vi "NI-DAQmxBase.vi"() -> (15 "error out":errorcluster)   [LabVIEW 2015]
uses:
  Globals/Meas_global.vi
  PWA/PWAtasksGLOBAL.vi
  <vilib>/_DAQmxBase/Internals/DAQmxBase Create Channel (AI-Voltage-Basic).vi
  <vilib>/_DAQmxBase/Internals/DAQmxBase Timing (Sample Clock).vi
  <vilib>/_DAQmxBase/Internals/DAQmxBase Read (Analog 2D DBL NChan NSamp).vi
  <resource>/objmgr/daqmx.rc
panel:
  out "AuditTrail":string[](array[string])
  out "input terminal configuration":i32(ring)=10106 items=["default"=-1, "RSE"=10083, "NRSE"=10078, "Differential"=10106, "Pseudodifferential"=12529]
  out "TotalSampPerChanAcquired":dbl=1024.0
  out "AvailSampPerChan":u32
  out "CurrReadPos":dbl=1024.0
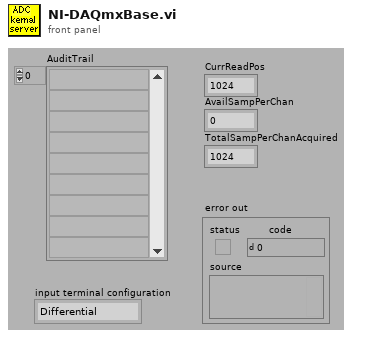
[diagram p1: front panel]
types:
  T1 = typedef "Ch_and_Spans.ctl" = cluster{"high limit (10V)":sgl, "low limit (-10V)":sgl, "Ch No":i16, "Var name":string, "Use Latest Calib":bool}
  T2 = typedef "LDA_Setup.ctl" = cluster{"dimensions":enum16{"1D", "2D"}, "Analogue Freq Multiplier":dbl}
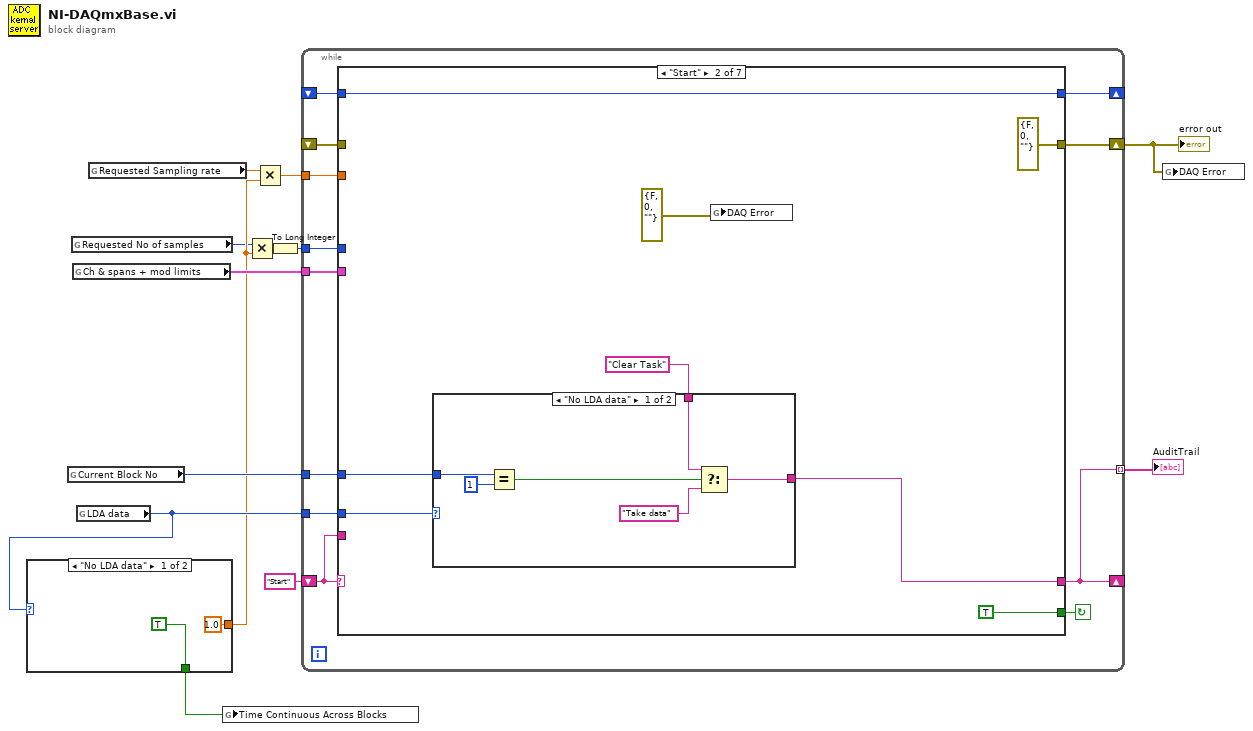
[diagram p0: block diagram]
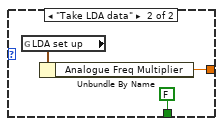
[diagram p2: hidden frame]
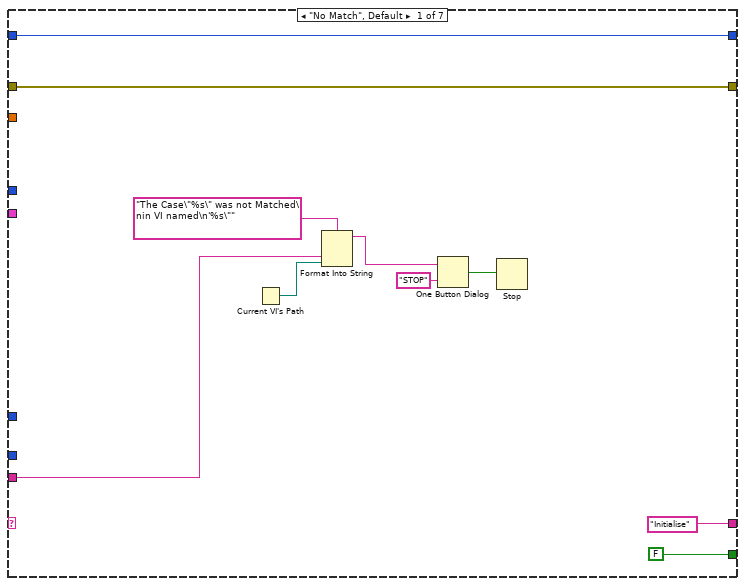
[diagram p3: hidden frame]
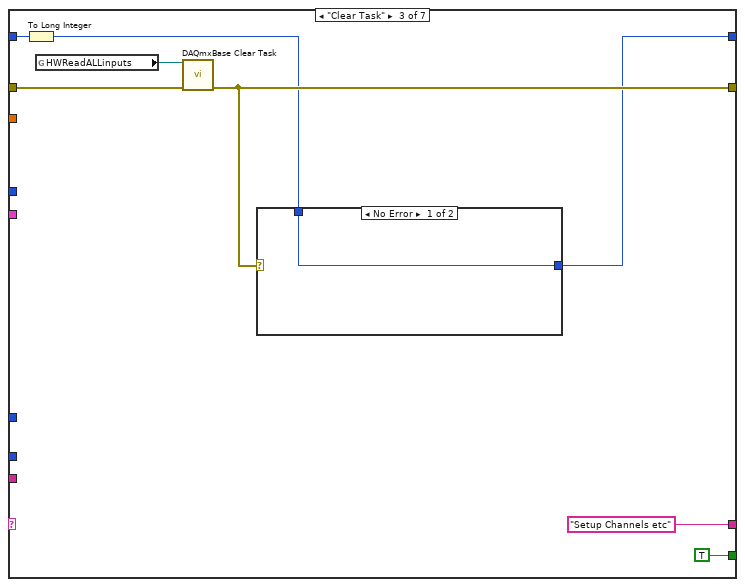
[diagram p5: hidden frame]
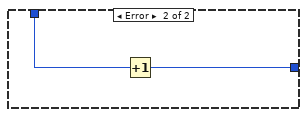
[diagram p6: hidden frame]
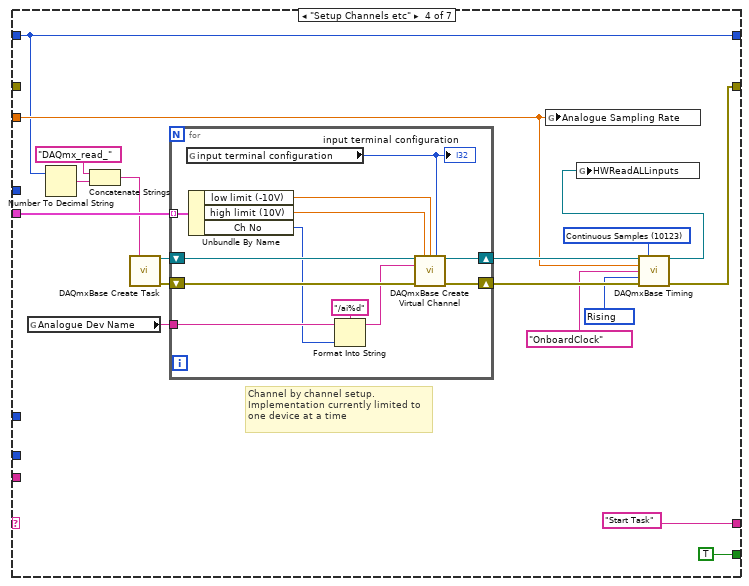
[diagram p7: hidden frame]
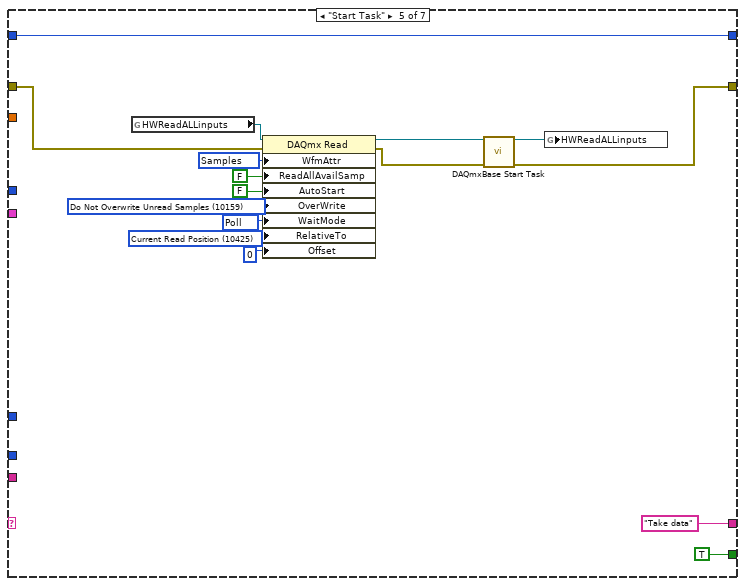
[diagram p8: hidden frame]
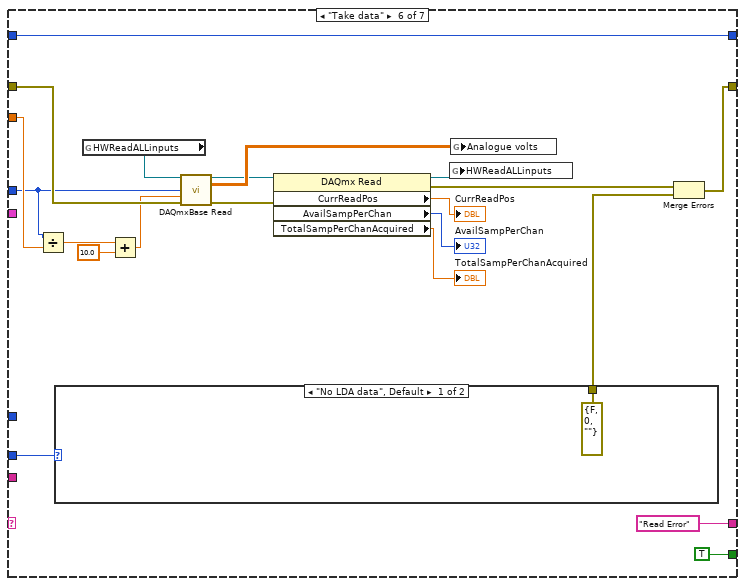
[diagram p9: hidden frame]
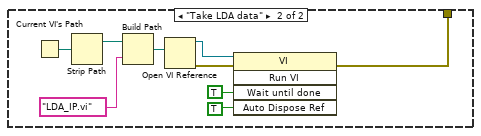
[diagram p10: hidden frame]
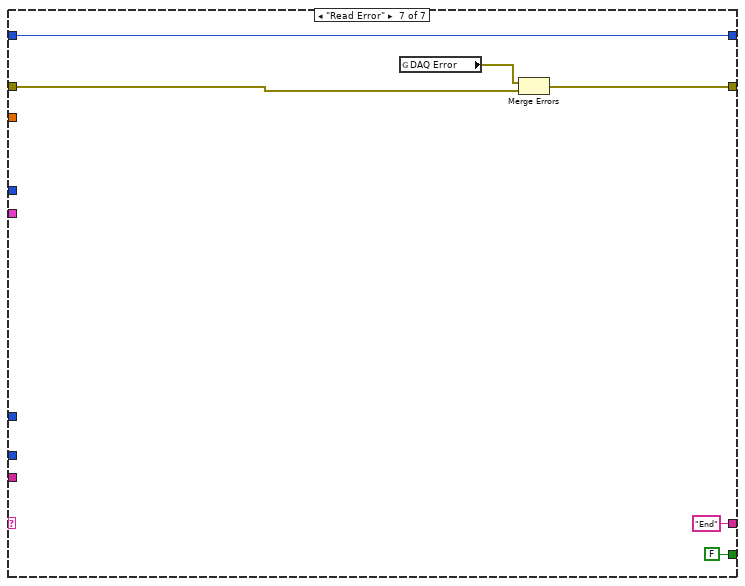
[diagram p11: hidden frame]
diagram:
  n1 = global read "Meas_global.vi" "Current Block No"() -> (w11:i32)
  n2 = global read "Meas_global.vi" "Requested No of samples"() -> (w1:i32)
  n3 = global read "Meas_global.vi" "Ch & spans + mod limits"() -> (w12:T1[])
  n4 = global read "Meas_global.vi" "LDA data"() -> (w9:enum16{"No LDA data", "Take LDA data"})
  n5 = case shown="\"No LDA data\"" w9 {
    tunnel: [1.0 ("Analogue Freq Multiplier") w17] -> w6
    tunnel: [TRUE ("Time Continuous across Blocks") FALSE ("Time Continuous across Blocks")] -> w2
    frame "No LDA data" {
    }
    frame "Take LDA data" {
      n6 = global read "Meas_global.vi" "LDA set up"() -> (w18:T2)
      n7 = Unbundle By Name(w18) -> ("Analogue Freq Multiplier"=w17:dbl)
    }
  }
  n8 = global read "Meas_global.vi" "Requested Sampling rate"() -> (w7:dbl)
  n9 = global write "Meas_global.vi" "Time Continuous Across Blocks"(w2) -> ()
  n10 = Multiply(x=w1, y=w6) -> (x*y=w8:dbl)
  n11 = Multiply(x=w7, y=w6) -> (x*y=w5:dbl)
  n12 = To Long Integer(number=w8) -> (32bit integer=w4:i32)
  n13 = while {
    shift-left: "Start" -> [w29]
    shift-right: [w19] -> _
    shift-right: [w23] -> w10
    shift-left: _ -> [w28]
    tunnel: w5 -> [w27]
    tunnel: w4 -> [w26]
    tunnel: w11 -> [w25]
    tunnel: w12 -> [w24]
    shift-right: [w22] -> _
    shift-left: _ -> [w21]
    tunnel: w9 -> [w20]
    tunnel: [w19] -> w3 mode=indexing
    stop <- w30 continue-if-true
    n14 = case shown="\"Start\"" w29 {
      tunnel: [FALSE TRUE TRUE TRUE TRUE TRUE FALSE] -> w30
      tunnel: ["Initialise" w46 "Setup Channels etc" "Start Task" "Take data" "Read Error" "End" ("f")] -> w19
      tunnel: w29 -> [w35 _ _ _ _ _ _]
      tunnel: [w32 errorcluster {"status"=FALSE, "code"=0, "source"=""} ("error out") w59 w78 w98 w115 w147] -> w23
      tunnel: w28 -> [w32 _ w60 _ w103 w133 w148]
      tunnel: w27 -> [_ _ _ w70 _ w123 _]
      tunnel: w26 -> [_ _ _ _ _ w114 _]
      tunnel: w25 -> [_ w43 _ _ _ _ _]
      tunnel: w24 -> [_ _ _ w77 _ _ _]
      tunnel: [w31 w45 w58 w69 w101 w124 w146] -> w22
      tunnel: w21 -> [w31 w45 w57 w69 w101 w124 w146]
      tunnel: w20 -> [_ w42 _ _ _ w118 _]
      frame "No Match", Default {
        n15 = Current VI's Path() -> (path=w34:path)
        n16 = Format Into String(format string="The Case\"%s\" was not Matched\nin VI named\n'%s\"" ("Format String"), w35, w34) -> (resulting string=w38:string)  [unwired: 2 in, 1 out]
        n17 = One Button Dialog(message=w38, button name ("OK")="STOP") -> (true=w36:bool)
        n18 = Stop(stop? (T)=w36) -> ()
      }
      frame "Start" {
        n19 = case shown="\"No LDA data\"" w42 {
          tunnel: "Clear Task" -> [w54 w55]
          tunnel: [w52 w55] -> w46
          tunnel: w43 -> [w51 _]
          frame "No LDA data" {
            n20 = Equal?(x=w51, y=1) -> (x = y?=w49:bool)
            n21 = Select(t=w54, s=w49, f="Take data") -> (s? t:f=w52:string)
          }
          frame "Take LDA data" {
          }
        }
        n22 = global write "Meas_global.vi" "DAQ Error"(errorcluster {"status"=FALSE, "code"=0, "source"=""} ("DAQ Error")) -> ()
      }
      frame "Clear Task" {
        n23 = To Long Integer(number=w57) -> (32bit integer=w56:i32)
        n24 = global read "PWAtasksGLOBAL.vi" "HWReadALLinputs"() -> (w61:refnum<k21>)
        n25 = call <vilib>:"DAQmxBase Clear Task.vi"("task in"=w61, "error in"=w60) -> ("error out"=w59:errorcluster)  [unwired: 13 in]
        n26 = case shown="No Error" w59 {
          tunnel: [w64 w65] -> w58
          tunnel: w56 -> [w64 w66]
          frame No Error {
          }
          frame Error {
            n27 = Increment(x=w66) -> (x+1=w65:i32)
          }
        }
      }
      frame "Setup Channels etc" {
        w76 = 10280 items=["Rising"=10280, "Falling"=10171] ("active edge")
        w81 = 10123 items=["Finite Samples"=10178, "Continuous Samples"=10123, "Hardware Timed Single Point"=12522] ("sample mode")
        # "Channel by channel setup. Implementation currently limited to one device at a time"
        n28 = global read "PWAtasksGLOBAL.vi" "Analogue Dev Name"() -> (w73:string)
        n29 = Number To Decimal String(number=w69) -> (decimal integer string=w68:string)  [unwired: 1 in]
        n30 = Concatenate Strings("DAQmx_read_" ("new task name"), w68) -> (w71:string)
        n31 = call <vilib>:"DAQmxBase Create Task.vi"("new task name"=w71) -> ("task out"=w79:refnum<k21>, "error out"=w82:errorcluster)  [unwired: 13 in]
        n32 = for {
          tunnel: w77 -> [w96] mode=indexing
          shift-right: [w94] -> w80
          shift-left: w79 -> [w95]
          shift-right: [w92] -> w83
          shift-left: w82 -> [w93]
          tunnel: w73 -> [w91]
          n33 = global read "Meas_global.vi" "input terminal configuration"() -> (w88:i32)
          "input terminal configuration" <- w88
          n34 = Unbundle By Name(w96) -> ("low limit (-10V)"=w87:sgl, "high limit (10V)"=w86:sgl, "Ch No"=w85:i16)
          n35 = Format Into String(format string="/ai%d", initial string=w91, w85) -> (resulting string=w89:string)  [unwired: 1 in, 1 out]
          n36 = call-poly <vilib>:"DAQmxBase Create Virtual Channel.vi"("task in"=w95, "maximum value"=w86, "minimum value"=w87, "input terminal configuration"=w88, "physical channels"=w89, "error in"=w93) -> ("task out"=w94:refnum<k21>, "error out"=w92:errorcluster)  [unwired: 8 in]
        }
        n37 = global write "Meas_global.vi" "Analogue Sampling Rate"(w70) -> ()
        n38 = call-poly <vilib>:"DAQmxBase Timing.vi"("task/channels in"=w80, "sample mode"=w81, "rate"=w70, "source"=tag "OnboardClock", "active edge"=w76, "error in"=w83) -> ("task out"=w67:refnum<k21>, "error out"=w78:errorcluster)  [unwired: 8 in]
        n39 = global write "PWAtasksGLOBAL.vi" "HWReadALLinputs"(w67) -> ()
      }
      frame "Start Task" {
        w106 = 10425 items=["First Sample"=10424, "Current Read Position"=10425, "Reference Trigger"=10426, "First Pretrigger Sample"=10427, "Most Recent Sample"=10428] ("RelativeTo")
        w107 = 12524 items=["Wait For Interrupt"=12523, "Poll"=12524, "Yield"=12525, "Sleep"=12547] ("WaitMode")
        w108 = 10159 items=["Overwrite Unread Samples"=10252, "Do Not Overwrite Unread Samples"=10159] ("OverWrite")
        w110 = 10287 items=["Samples"=10287, "Samples and Timing"=10140, "Samples, Timing, and Attributes"=10141] ("WfmAttr")
        n40 = global read "PWAtasksGLOBAL.vi" "HWReadALLinputs"() -> (w104:refnum<k21>)
        n41 = property class="DAQmx Read"(reference=w104, error in=w103, "WfmAttr"=w110, "ReadAllAvailSamp"=FALSE, "AutoStart"=FALSE, "OverWrite"=w108, "WaitMode"=w107, "RelativeTo"=w106, "Offset"=0) -> (reference out=w99:refnum<k21>, error out=w100:errorcluster)
        n42 = call <vilib>:"DAQmxBase Start Task.vi"("task/channels in"=w99, "error in"=w100) -> ("task out"=w97:refnum<k21>, "error out"=w98:errorcluster)  [unwired: 12 in]
        n43 = global write "PWAtasksGLOBAL.vi" "HWReadALLinputs"(w97) -> ()
      }
      frame "Take data" {
        n44 = Divide(x=w114, y=w123) -> (x/y=w122:dbl)
        n45 = case shown="\"No LDA data\", Default" w118 {
          tunnel: [errorcluster {"status"=FALSE, "code"=0, "source"=""} ("error out") w135] -> w117
          frame "No LDA data", Default {
          }
          frame "Take LDA data" {
            n46 = Current VI's Path() -> (path=w137:path)
            n47 = Strip Path(path=w137) -> (stripped path=w136:path)  [unwired: 1 out]
            n48 = Build Path(base path=w136, name or relative path="LDA_IP.vi") -> (appended path=w138:path)
            n49 = Open VI Reference(vi path=w138) -> (vi reference=w141:refnum<vi>, error out=w142:errorcluster)  [unwired: 5 in]
            n50 = invoke class="VI" method="Run VI"(reference=w141, error in=w142, "Wait until done"=TRUE ("Wait Until Done"), "Auto Dispose Ref"=TRUE ("Wait until done")) -> (error out=w135:errorcluster)  [unwired: 1 in, 4 out]
          }
        }
        n51 = global read "PWAtasksGLOBAL.vi" "HWReadALLinputs"() -> (w127:refnum<k21>)
        n52 = Add(x=w122, y=10.0) -> (x+y=w120:dbl)
        n53 = call-poly <vilib>:"DAQmxBase Read.vi"("task/channels in"=w127, "number of samples per channel"=w114, "timeout"=w120, "error in"=w133) -> ("task out"=w113:refnum<k21>, "data"=w119:dbl[][], "error out"=w126:errorcluster)  [unwired: 9 in]
        n54 = property class="DAQmx Read"(reference=w113, error in=w126) -> (reference out=w130:refnum<k21>, error out=w116:errorcluster, "CurrReadPos"=→"CurrReadPos":dbl, "AvailSampPerChan"=→"AvailSampPerChan":u32, "TotalSampPerChanAcquired"=→"TotalSampPerChanAcquired":dbl)
        n55 = global write "PWAtasksGLOBAL.vi" "HWReadALLinputs"(w130) -> ()
        n56 = global write "Meas_global.vi" "Analogue volts"(w119) -> ()
        n57 = Merge Errors(w116, w117) -> (w115:errorcluster)
      }
      frame "Read Error" {
        n58 = global read "Meas_global.vi" "DAQ Error"() -> (w149:errorcluster)
        n59 = Merge Errors(w149, w148) -> (w147:errorcluster)
      }
    }
  }
  "error out" <- w10
  "AuditTrail" <- w3
  n60 = global write "Meas_global.vi" "DAQ Error"(w10) -> ()
